vi "oax_Set IEPE & Coupling.vi"(8 "error in (no error)":errorcluster, 10 "DAQ Config":T1 {"pregain" format="%.2f"; "IEPE" items=["On", "Off", "None"]; "coupling" items=["DC", "AC"]; "engineering units" items=["custom..."=0, "V"=1, "A"=21, "C"=30, "pC"=31, "s"=32, "-"=29, "Pa"=2, "N"=20, "g"=3, "m/s^2"=4, "m/s"=5, "m"=6, "mm/s"=12, "mm"=13, "micron/s"=14, "micron"=15, "in/s^2"=7, "in/s"=8, "in"=9, "mil/s"=10, "mil"=11, "rad/s^2"=16, "rad/s"=17, "rad"=18, "deg/s^2"=26, "deg/s"=27, "deg"=28, "RPM"=22, "cycle/s^2"=23, "Hz"=24, "cycle"=25, "strain"=19]; "sensor sensitivity (mV/EU)" format="%.2f"; "dB reference" format="%.1e"}, 11 "task in":refnum<k21>) -> (0 "error out":errorcluster, 3 "task out":refnum<k21>)   [LabVIEW 2017]
uses:
  <vilib>/addons/Sound and Vibration/Order Analysis/Example Support/sub VIs/OAXML_DSA DAQ Config.ctl
  <vilib>/addons/_NISVFA/_Shared subVIs/Controls/svc_Engineering Units Text Ring.ctl
  <resource>/objmgr/daqmx.rc
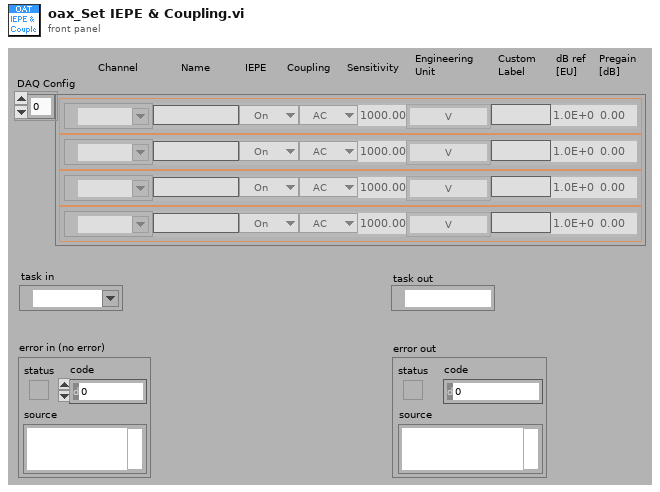
[diagram p1: front panel]
types:
  T1 = typedef "OAXML_DSA DAQ Config.ctl" = cluster{"name":string, "channel":tag, "coupling":u16, "dB reference":sgl, "sensor sensitivity (mV/EU)":dbl, "engineering units":T2, "IEPE":u16, "custom label":string, "pregain":sgl}[]
  T2 = typedef "svc_Engineering Units Text Ring.ctl" = u16
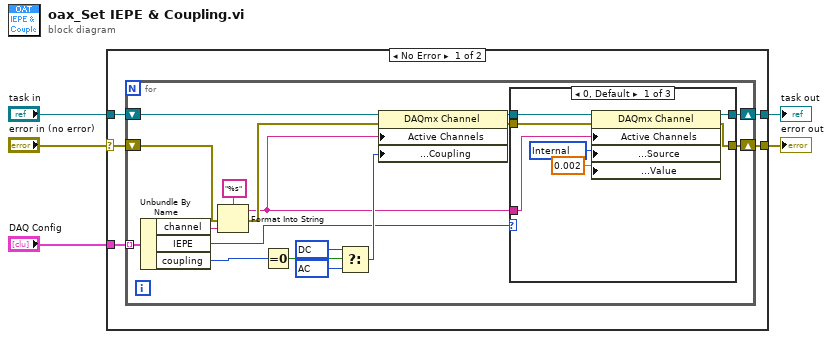
[diagram p0: block diagram]
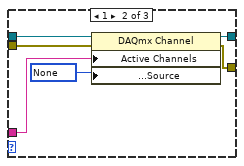
[diagram p2: hidden frame]
diagram:
  n1 = case shown="No Error" "error in (no error)" {
    selector: "error in (no error)" -> [w8 w43]
    tunnel: "task in" -> [w9 w44]
    tunnel: "DAQ Config" -> [w10 _]
    tunnel: [w7 w44] -> w2
    tunnel: [w6 w43] -> w1
    frame No Error {
      n2 = for {
        tunnel: w10 -> [w27] mode=indexing
        shift-right: [w12] -> w7
        shift-left: w9 -> [w24]
        shift-right: [w11] -> w6
        shift-left: w8 -> [w23]
        w19 = 10045 items=["AC"=10045, "DC"=10050, "GND"=10066] ("AI.Coupling")
        w17 = 10050 items=["AC"=10045, "DC"=10050, "GND"=10066] ("AI.Coupling")
        n3 = Unbundle By Name(w27) -> ("channel"=w26:tag, "IEPE"=w14:u16, "coupling"=w21:u16)
        n4 = Format Into String(format string="%s", error in=w23, w26) -> (resulting string=w13:string, error out=w22:errorcluster)  [unwired: 1 in]
        n5 = Equal To 0?(x=w21) -> (x = 0?=w20:bool)
        n6 = Select(t=w17, s=w20, f=w19) -> (s? t:f=w18:i32)
        n7 = property class="DAQmx Channel"(reference=w24, error in=w22, "Active Channels"=w13, "Analog Input:General Properties:Input Configuration:Coupling"=w18) -> (reference out=w16:refnum<k21>, error out=w15:errorcluster)
        n8 = case shown="0, Default" w14 {
          tunnel: w16 -> [w32 w39 w42]
          tunnel: w15 -> [w30 w37 w41]
          tunnel: w13 -> [w28 w35 _]
          tunnel: [w31 w38 w42] -> w12
          tunnel: [w29 w36 w41] -> w11
          frame 0, Default {
            w34 = 10200 items=["Internal"=10200, "External"=10167, "None"=10230] ("AI.Excit.Src")
            n9 = property class="DAQmx Channel"(reference=w32, error in=w30, "Active Channels"=w28, "Analog Input:General Properties:Signal Conditioning:Excitation:Source"=w34, "Analog Input:General Properties:Signal Conditioning:Excitation:Value"=0.002 ("AI.Excit.Val")) -> (reference out=w31:refnum<k21>, error out=w29:errorcluster)
          }
          frame 1 {
            w40 = 10230 items=["Internal"=10200, "External"=10167, "None"=10230] ("AI.Excit.Src")
            n10 = property class="DAQmx Channel"(reference=w39, error in=w37, "Active Channels"=w35, "Analog Input:General Properties:Signal Conditioning:Excitation:Source"=w40) -> (reference out=w38:refnum<k21>, error out=w36:errorcluster)
          }
          frame 2 {
          }
        }
      }
    }
    frame Error {
    }
  }
  "task out" <- w2
  "error out" <- w1
